vi "Initialize.vi"(7 "ChannelName":string="Setpoint.ch%d.SP", 8 "error in":errorcluster, 9 "Number of Channels":u32=1, 10 "Plugin Name":string, 11 "Capabilities in":refnum<class "Capabilities.lvclass">) -> (0 "error out":errorcluster, 3 "Capabilities out":refnum<class "Capabilities.lvclass">)   [LabVIEW 2023, in "Capabilities.lvclass"]
uses:
  Capabilities.lvclass
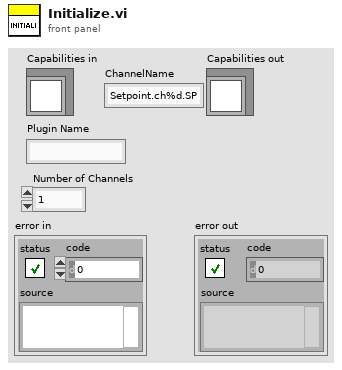
[diagram p1: front panel]
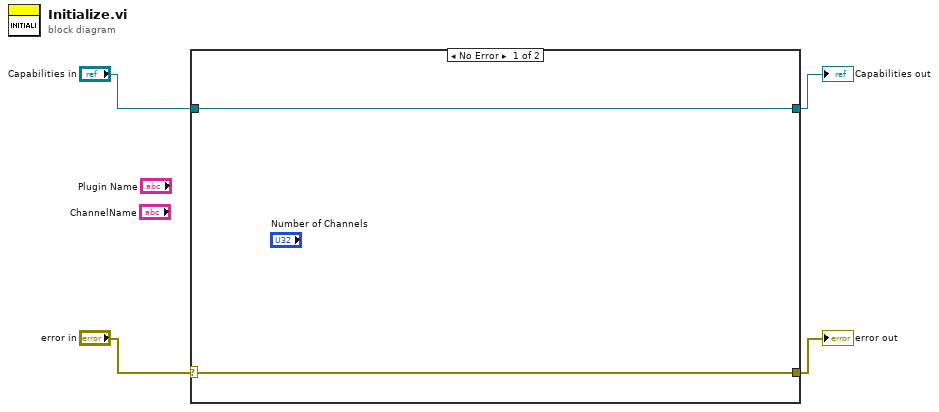
[diagram p0: block diagram]
diagram:
  n1 = case shown="No Error" "error in" {
    selector: "error in" -> [w5 w8]
    tunnel: [w5 w8] -> w1
    tunnel: [w6 w7] -> w3
    tunnel: "Capabilities in" -> [w6 w7]
    frame No Error {
    }
    frame Error {
    }
  }
  "error out" <- w1
  "Capabilities out" <- w3
